vi "fgv_lidar-range_vh.vi"(7 "cmd":enum16{"read", "write"}(ring), 11 "VLP16 cfg":T1={"h range"={82, -88}, "v range"={7, -9}} {"v range" scale=-15.0..15.0; "h range" scale=-180.0..180.0}) -> (3 "VLP16 cfg out":T1={"h range"={0, 9}, "v range"={0, 9}} {"v range" scale=-15.0..15.0; "h range" scale=-180.0..180.0})   [LabVIEW 2019]
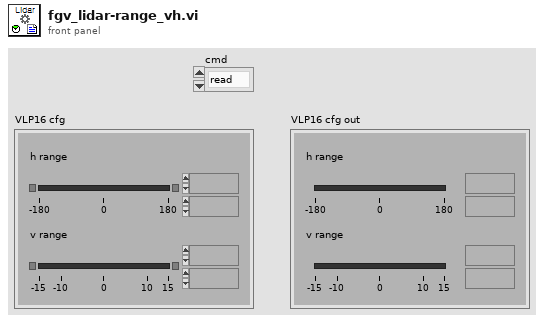
[diagram p1: front panel]
types:
  T1 = cluster{"h range":cluster{i16, i16}, "v range":cluster{i8, i8}}
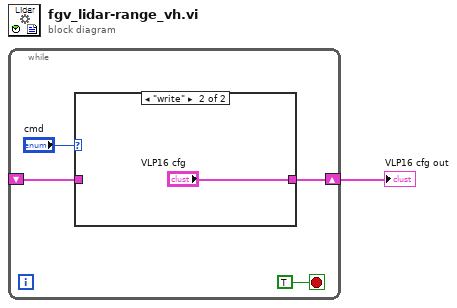
[diagram p0: block diagram]
diagram:
  n1 = while {
    shift-right: [w3] -> w1
    shift-left: _ -> [w2]
    stop <- TRUE stop-if-true
    n2 = case shown="\"write\"" "cmd" {
      tunnel: [w6 "VLP16 cfg"] -> w3
      tunnel: w2 -> [w6 _]
      frame "read", Default {
      }
      frame "write" {
      }
    }
  }
  "VLP16 cfg out" <- w1
